vi "Main v0.4.vi"() -> ()   [LabVIEW 2017]
doc: "This template is for the Queued Message Handler design pattern.\n\nThe Event Handling Loop generates messages based on user interface actions.\n\nThe Message Handling Loop processes messages generated by the Event Handling Loop, or by other messages. The messages are string values, so new messages can be added easily to the Message Cases case structure in the Message Handling Loop. Each message cluster can also provide an optional value for Message Data, which is a variant that can be converted to whatever message-specific data is required."
uses:
  Controls/Main Tabs.ctl
  Controls/Auto.ctl
  RT/Controls/Auto Delays.ctl
  RT/Controls/Auto Times.ctl
  <userlib>/SESL Controls/refresh ES.ctl
  Controls/UI Data.ctl
  support/Message Queue/Enqueue Message (Single).vi
  <vilib>/Utility/error.llb/Error Cluster From Error Code.vi
  <vilib>/ErrorRing/Error Ring.xnode
  support/Message Queue/Message Queue.lvlib
  support/User Event - Stop/User Event - Stop.lvlib
panel:
  in  "Enable Reject?":bool
  out "Date-Time":string caption="Dip-Tube Assembly Automation (HMI) v0.4"
  out "Main Tab":T1
  in  "Autocycle":T2
  in  "Manual":bool
  in  "Parameters":bool
  in  "Maintenance":bool
  in  "Save Para":bool
  in  "Home Para":bool
  in  "ParaTab":T3(tab)
  in  "StopperRearDelay":dbl format="%#.2f"
  in  "StopperFrontDelay":dbl format="%#.2f"
  in  "MaxAlarms":dbl caption="Max Alarms in 1 Minute" format="%#.2f"
  in  "MaxConsecutive":dbl caption="Max Consecutive Alarms" format="%#.2f"
  in  "Gate Close Delay":dbl format="%#.2f"
  in  "Gate Open Delay":dbl format="%#.2f"
  in  "BF Off Delay":dbl format="%#.2f"
  in  "BF On Delay":dbl format="%#.2f"
  in  "DelayAfterReject":dbl format="%#.2f"
  in  "MeasurementTime":dbl format="%#.2f"
  in  "DelayAfterMesFront":dbl format="%#.2f"
  in  "DelayAfterCut":dbl format="%#.2f"
  in  "DelayAfterCutClamp":dbl format="%#.2f"
  in  "DelayAfterInsClamp":dbl format="%#.2f"
  in  "DelayToClose":dbl format="%#.2f"
  in  "DelayToOpen":dbl format="%#.2f"
  in  "DelayAfterInsertion":dbl format="%#.2f"
  in  "DelayBeforeInsertion":dbl format="%#.2f"
  in  "AgitatorUpTime":dbl format="%#.2f"
  in  "AgitatorDownTime":dbl format="%#.2f"
  in  "Toggle Motor":bool
  in  "Continuous?":T4
  in  "Enable Measure?":bool
  in  "Enable Index?":bool
  in  "Enable PF?":bool
  in  "Auto Delays":T5={"Agitator Delays"=[1000], "TF Delays"=[1000], "Insertion Delays"=[1000, 1000], "Cutting Delays"=[1000, 1000, 1000], "PF Delays"=[1000], "Measur. Delays"=[1000]}
  in  "Enable Cutting?":bool
  in  "Enable Insertion?":bool
  in  "Run Manual":bool
  in  "Enable TF?":bool
  in  "Home Manual":bool
  out "Status":T7
  out "Measurements":cluster{"1":dbl, "2":dbl, "3":dbl, "4":dbl} {"1" format="%#.2f"; "2" format="%#.2f"; "3" format="%#.2f"; "4" format="%#.2f"}
  in  "All IO":bool
  in  "Stats":bool
  in  "Home AC":bool
  out "Status":string
  out "Count":dbl format="%06.0f"
  out "Count 3":dbl caption="Cycle Time" format="%0.2f"
  out "Count 2":dbl caption="Rejects" format="%06.0f"
  in  "Statuses":string[][](table)
  in  "Exit":bool
  # "Vision Harmony Dip-Tube Assembly Automation"
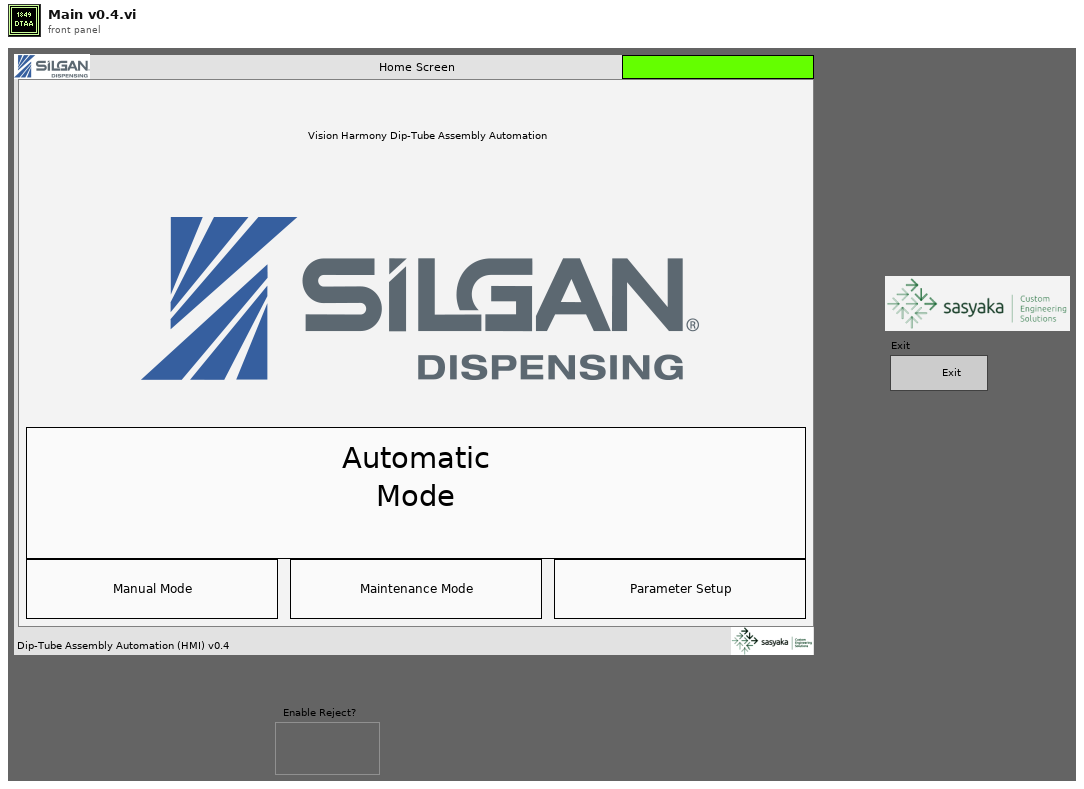
[diagram p1: front panel]
types:
  T1 = typedef "Main Tabs.ctl" = enum32{"Home Screen", "Parameter Setup", "Manual Mode", "Autocycle"}
  T2 = typedef "Auto.ctl" = bool
  T3 = enum32{"General & Indexing", "Bowl Feeder & Pump Conveyor", "Cutting, Measurement & Rejection", "Tube Feeder & Insertion"}
  T4 = typedef "refresh ES.ctl" = bool
  T5 = typedef "Auto Delays.ctl" = cluster{"Agitator Delays":u32[], "TF Delays":u32[], "Insertion Delays":u32[], "Cutting Delays":u32[], "PF Delays":u32[], "Measur. Delays":u32[]}
  T6 = typedef "Auto Times.ctl" = cluster{"Index Time":u32, "TF Time":u32, "Insertion Time":u32, "Cutting Time":u32, "PF Time":u32, "Meas. Time":u32}
  T7 = cluster{"Auto Times":T6, "error out":errorcluster}
  T8 = typedef "UI Data.ctl" = cluster{"Main Tab":refnum<vi>}
  T9 = typedef "Message Queue.lvlib/All Message Queues.ctl" = cluster{"UI":refnum<queue>}
  T10 = enum8{"Enabled", "Disabled", "Disabled and Grayed Out"}
  T11 = cluster{"Auto Times":T6, "Measurements":cluster{"1":dbl, "2":dbl, "3":dbl, "4":dbl}, "error out":errorcluster}
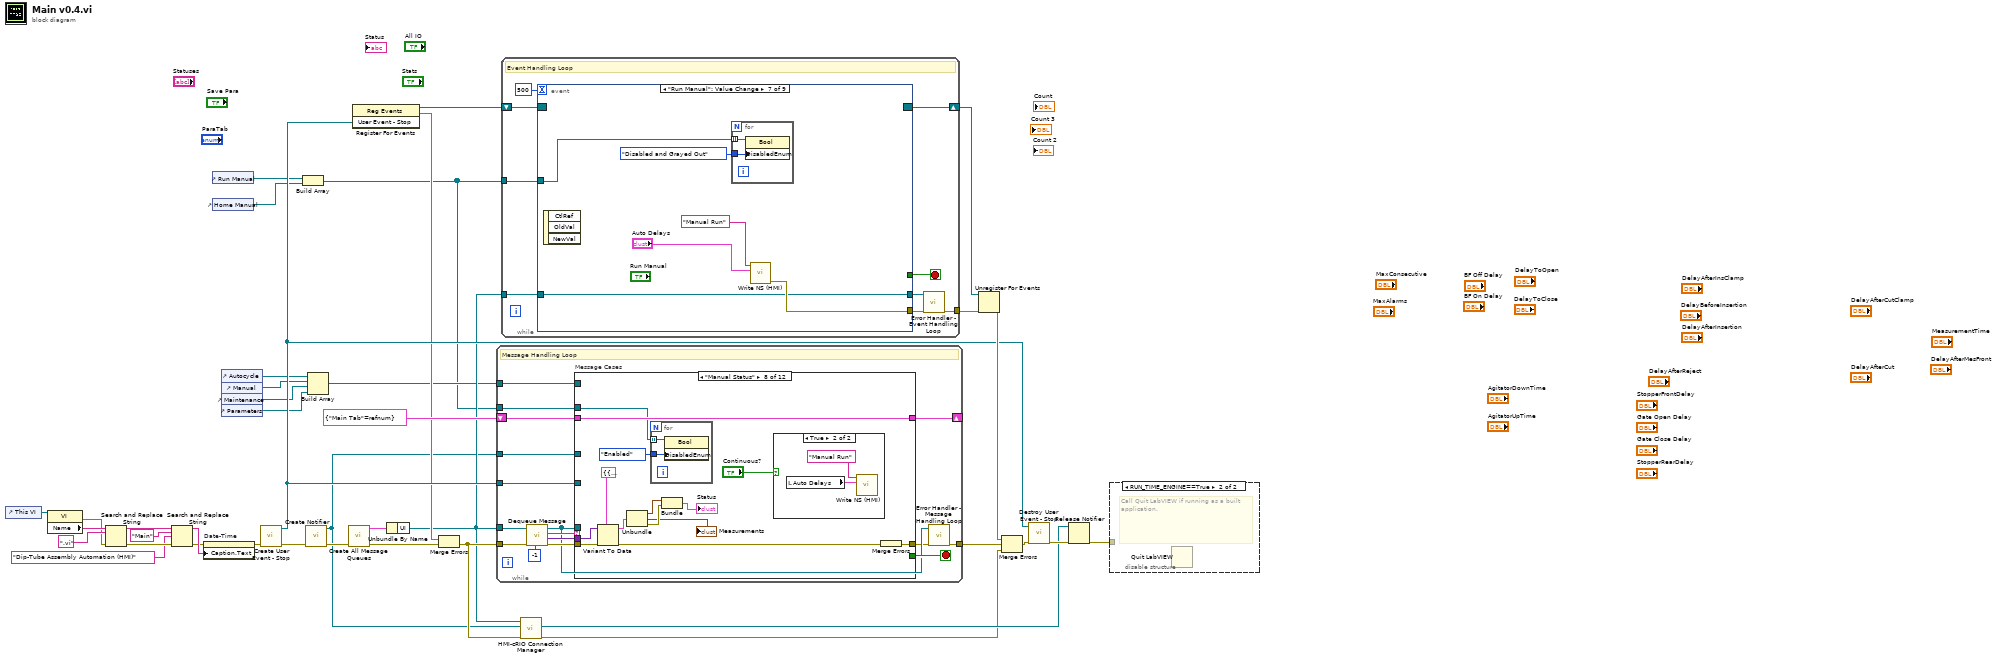
[diagram p0: block diagram]
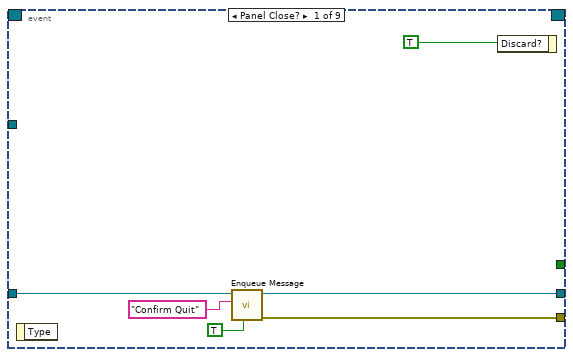
[diagram p2: hidden frame]
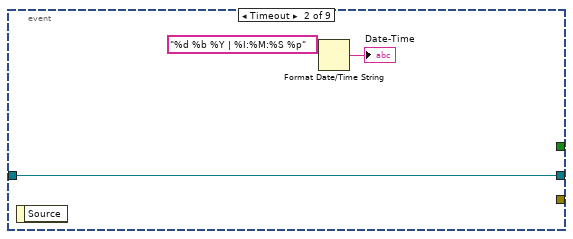
[diagram p3: hidden frame]
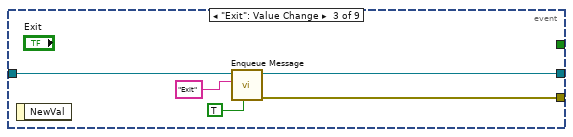
[diagram p4: hidden frame]
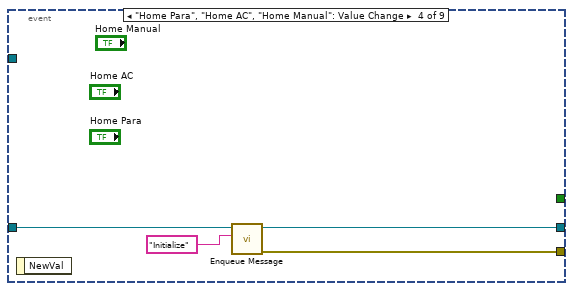
[diagram p5: hidden frame]
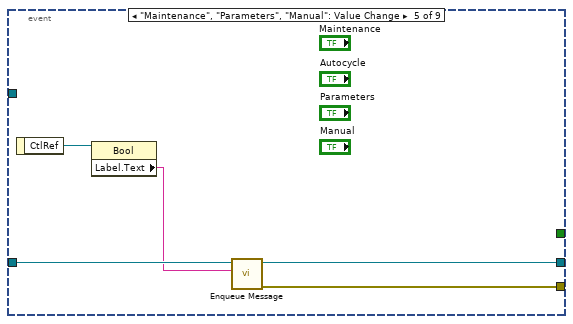
[diagram p6: hidden frame]
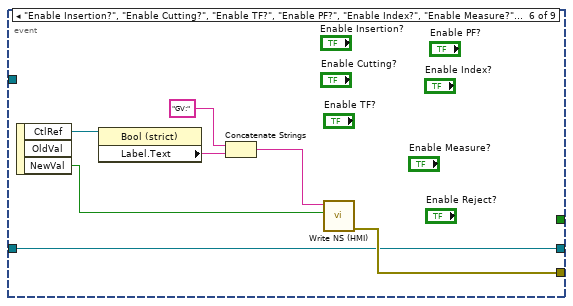
[diagram p7: hidden frame]
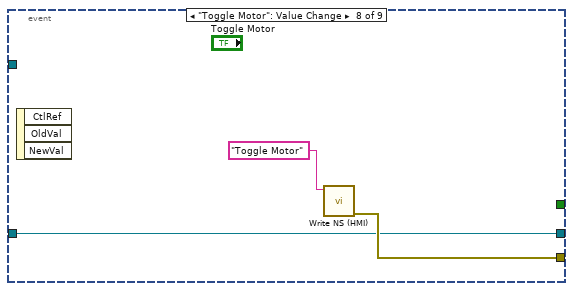
[diagram p8: hidden frame]
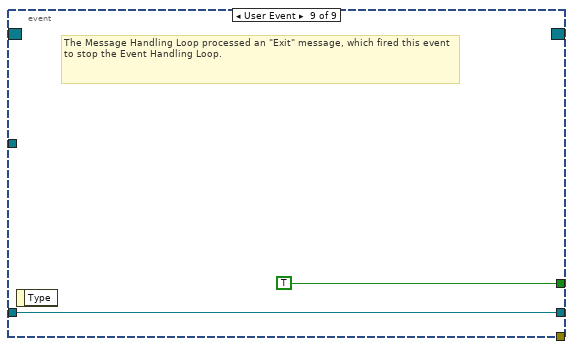
[diagram p9: hidden frame]
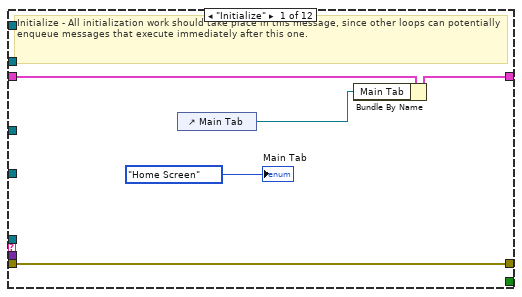
[diagram p10: hidden frame]
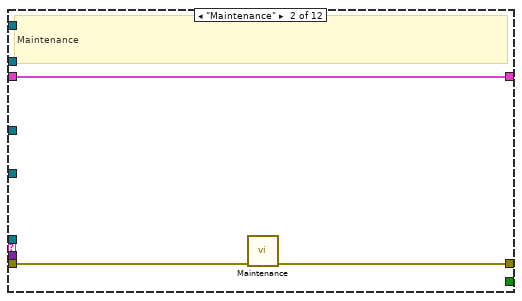
[diagram p11: hidden frame]
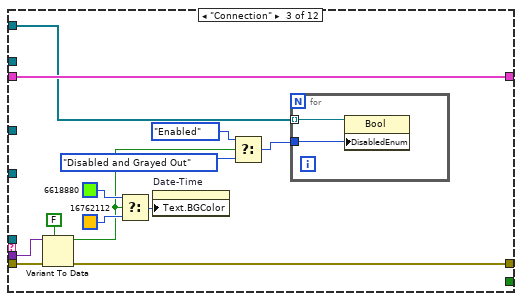
[diagram p12: hidden frame]
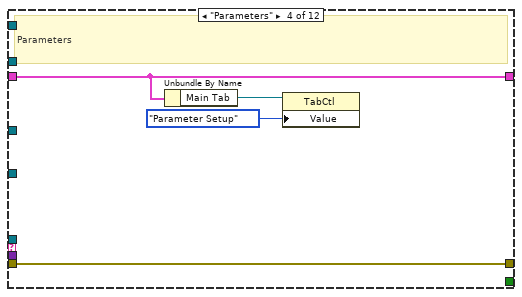
[diagram p13: hidden frame]
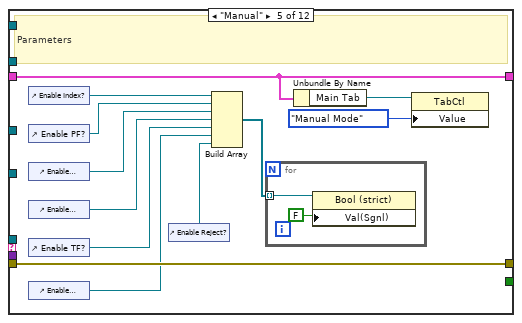
[diagram p14: hidden frame]
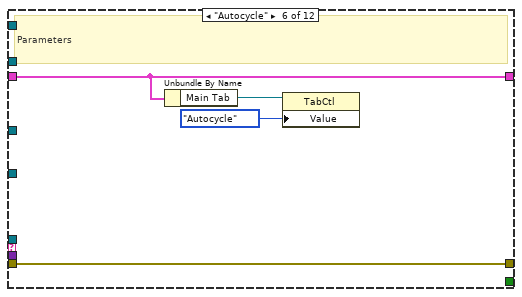
[diagram p15: hidden frame]
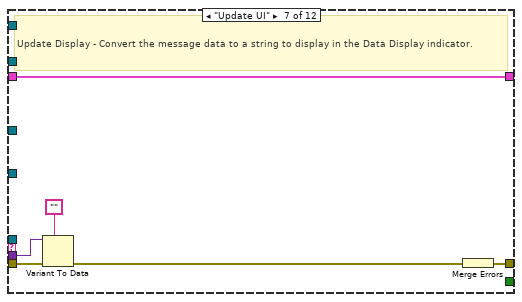
[diagram p16: hidden frame]
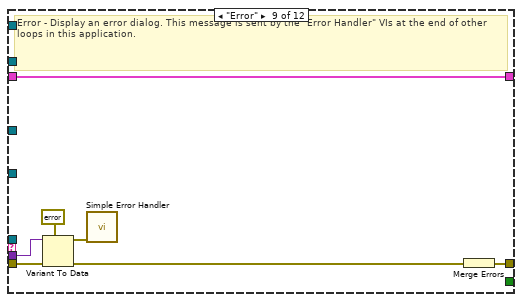
[diagram p18: hidden frame]
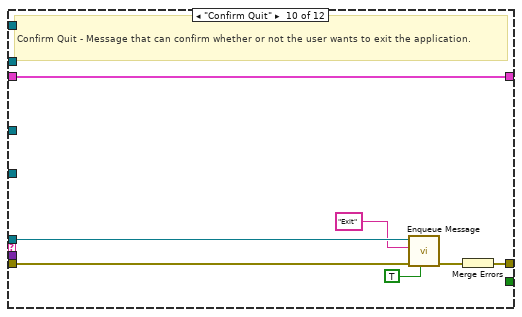
[diagram p19: hidden frame]
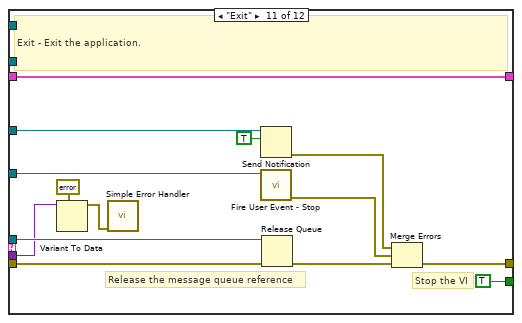
[diagram p20: hidden frame]
diagram:
  n1 = control-ref of="This VI"() -> (w8:refnum<vi>)
  n2 = property class="VI"(reference=w8) -> (error out=w7:errorcluster, "Name"=w14:string)  [unwired: 1 in, 1 out]
  n3 = Search and Replace String(input string=w14, search string=".vi", error in=w7) -> (result string=w12:string, error out=w11:errorcluster)  [unwired: 5 in, 2 out]
  n4 = Search and Replace String(input string=w12, search string="Main", replace string="Dip-Tube Assembly Automation (HMI)" ("replace string (\"\")"), error in=w11) -> (result string=w6:string, error out=w5:errorcluster)  [unwired: 4 in, 2 out]
  n5 = property on="Date-Time" class="Str"(error in=w5, "Caption.Text"=w6) -> (error out=w4:errorcluster)  [unwired: 1 in, 1 out]
  n6 = control-ref of="Run Manual"() -> (w3:refnum<vi>)
  n7 = control-ref of="Home Manual"() -> (w2:refnum<vi>)
  n8 = control-ref of="Autocycle"() -> (w19:refnum<vi>)
  n9 = control-ref of="Manual"() -> (w18:refnum<vi>)
  n10 = control-ref of="Maintenance"() -> (w17:refnum<vi>)
  n11 = control-ref of="Parameters"() -> (w16:refnum<vi>)
  n12 = call "Create User Event - Stop.vi"("error in (no error)"=w4) -> ("error out"=w26:errorcluster, "User Event - Stop"=w30:refnum<user-event>)  [unwired: 9 in]
  n13 = Build Array(w3, w2) -> (w1:refnum<vi>[])
  n14 = call "Create Notifier.vi"("error in (no error)"=w26) -> ("error out"=w25:errorcluster, "notifier out"=w20:refnum<notifier>)  [unwired: 9 in]
  n15 = Build Array(w19, w18, w17, w16) -> (w15:refnum<vi>[])
  n16 = call "Create All Message Queues.vi"("error in (no error)"=w25) -> ("error out"=w39:errorcluster, "Message Queues out"=w38:T9)  [unwired: 9 in]
  n17 = register-events(w30) -> (reference out=w31:refnum<event-registration>, error out=w29:errorcluster)  [unwired: 2 in]
  n18 = Unbundle By Name(w38) -> ("UI"=w27:refnum<queue>)
  n19 = Merge Errors(w29, w39) -> (w28:errorcluster)
  n20 = while {
    tunnel: w27 -> [w47]
    shift-right: [w54] -> _
    shift-left: T8 {"Main Tab"=refnum} ("Data Cluster") -> [w55]
    tunnel: w30 -> [w52]
    tunnel: w28 -> [w51]
    tunnel: [w45] -> w37
    tunnel: w20 -> [w42]
    tunnel: w15 -> [w41]
    tunnel: w1 -> [w40]
    stop <- w53 stop-if-true
    # "Message Handling Loop"
    n21 = call "Dequeue Message.vi"("timeout"=-1, "error in (no error)"=w51, "Message Queue"=w47) -> ("error out"=w50:errorcluster, "Message Data"=w48:variant, "Message"=w49:string, "dup Message Queue"=w46:refnum<queue>)  [unwired: 5 in]
    n22 = case "Message Cases" shown="\"Manual Status\"" w49 {
      selector: w49 -> [_ _ _ _ _ _ _ _ _ _ _ w153]
      tunnel: w46 -> [_ _ _ _ _ _ _ _ _ w134 w152 _]
      tunnel: w50 -> [w60 w62 w74 w82 w94 w100 w104 w118 w131 w138 w145 _]
      tunnel: [w60 w61 w73 w82 w94 w100 w105 w119 w125 w136 w148 w154] -> w44
      tunnel: w55 -> [w59 w63 w76 w81 w93 w99 w106 w120 w130 w137 w151 w155]
      tunnel: [w58 w63 w76 w81 w93 w99 w106 w120 w130 w137 w151 w155] -> w54
      tunnel: [_ _ _ _ _ _ _ _ _ _ TRUE _] -> w53
      tunnel: w48 -> [_ _ w72 _ _ _ w103 w117 w129 _ w142 _]
      tunnel: w52 -> [_ _ _ _ _ _ _ _ _ _ w147 _]
      tunnel: w42 -> [_ _ _ _ _ _ _ _ _ _ w141 _]
      tunnel: w41 -> [_ _ w68 _ _ _ _ _ _ _ _ _]
      tunnel: w40 -> [_ _ _ _ _ _ _ w114 _ _ _ _]
      frame "Initialize" {
        # "Initialize - All initialization work should take place in this message, since other loops can potentially enqueue messages that execute immediately after this one."
        n23 = control-ref of="Main Tab"() -> (w57:refnum<vi>)
        n24 = Bundle By Name(cluster=w59, "Main Tab"=w57) -> (w58:T8)
        "Main Tab" <- Main_Tabs."Home Screen" ("Main Tab")
      }
      frame "Maintenance" {
        # "Maintenance"
        n25 = call "Maintenance.vi"("Error In"=w62) -> ("Error out"=w61:errorcluster)  [unwired: 10 in]
      }
      frame "Connection" {
        n26 = Variant To Data(error in=w74, type=FALSE, Variant=w72) -> (data=w67:bool, error out=w73:errorcluster)
        n27 = Select(t=u32 6618880 ("Text.Text Colors:BG Color"), s=w67, f=u32 16762112 ("Text.Text Colors:BG Color")) -> (s? t:f=w69:u32)
        n28 = property on="Date-Time" class="Str"("Text.BGColor"=w69) -> ()  [unwired: 2 in, 2 out]
        n29 = Select(t=T10."Enabled" ("Disabled"), s=w67, f=T10."Disabled and Grayed Out") -> (s? t:f=w65:T10)
        n30 = for {
          tunnel: w68 -> [w78] mode=indexing
          tunnel: w65 -> [w77]
          n31 = property class="Bool"(reference=w78, "DisabledEnum"=w77) -> ()  [unwired: 1 in, 2 out]
        }
      }
      frame "Parameters" {
        # "Parameters"
        n32 = Unbundle By Name(w81) -> ("Main Tab"=w80:refnum<vi>)
        n33 = property class="TabCtl"(reference=w80, "Value"=Main_Tabs."Parameter Setup" ("Main Tab")) -> ()  [unwired: 1 in, 2 out]
      }
      frame "Manual" {
        # "Parameters"
        n34 = control-ref of="Enable Index?"() -> (w90:refnum<vi>)
        n35 = control-ref of="Enable PF?"() -> (w89:refnum<vi>)
        n36 = control-ref of="Enable Cutting?"() -> (w88:refnum<vi>)
        n37 = control-ref of="Enable Insertion?"() -> (w87:refnum<vi>)
        n38 = control-ref of="Enable TF?"() -> (w86:refnum<vi>)
        n39 = control-ref of="Enable Measure?"() -> (w84:refnum<vi>)
        n40 = control-ref of="Enable Reject?"() -> (w83:refnum<vi>)
        n41 = Build Array(w90, w89, w88, w87, w86, w84, w83) -> (w85:refnum<vi>[])
        n42 = for {
          tunnel: w85 -> [w96] mode=indexing
          n43 = property class="Bool (strict)"(reference=w96, "Val(Sgnl)"=FALSE ("Value (Signaling)")) -> ()  [unwired: 1 in, 2 out]
        }
        n44 = Unbundle By Name(w93) -> ("Main Tab"=w92:refnum<vi>)
        n45 = property class="TabCtl"(reference=w92, "Value"=Main_Tabs."Manual Mode" ("Main Tab")) -> ()  [unwired: 1 in, 2 out]
      }
      frame "Autocycle" {
        # "Parameters"
        n46 = Unbundle By Name(w99) -> ("Main Tab"=w98:refnum<vi>)
        n47 = property class="TabCtl"(reference=w98, "Value"=Main_Tabs."Autocycle" ("Main Tab")) -> ()  [unwired: 1 in, 2 out]
      }
      frame "Update UI" {
        # "Update Display - Convert the message data to a string to display in the Data Display indicator."
        n48 = Variant To Data(error in=w104, type="", Variant=w103) -> (error out=w101:errorcluster)  [unwired: 1 out]
        n49 = Merge Errors(w101) -> (w105:errorcluster)
      }
      frame "Manual Status" {
        n50 = Variant To Data(error in=w118, type=T11 {"Auto Times"={"Index Time"=0, "TF Time"=0, "Insertion Time"=0, "Cutting Time"=0, "PF Time"=0, "Meas. Time"=0}, "Measurements"={"1"=0.0, "2"=0.0, "3"=0.0, "4"=0.0}, "error out"={"status"=FALSE, "code"=0, "source"=""}} ("cluster"), Variant=w117) -> (data=w112:T11, error out=w116:errorcluster)
        n51 = Unbundle(w112) -> ("Auto Times"=w111:T6, "Measurements"=→"Measurements":cluster{"1":dbl, "2":dbl, "3":dbl, "4":dbl}, "error out"=w110:errorcluster)
        n52 = for {
          tunnel: w114 -> [w124] mode=indexing
          tunnel: T10."Enabled" ("Disabled") -> [w123]
          n53 = property class="Bool"(reference=w124, "DisabledEnum"=w123) -> ()  [unwired: 1 in, 2 out]
        }
        n54 = Bundle("Auto Times"=w111, "error out"=w110) -> (→"Status":T7)  [unwired: 1 in]
        n55 = case shown="True" "Continuous?" {
          frame False {
          }
          frame True {
            n56 = local read "Auto Delays"() -> (w121:T5)
            n57 = call "Write NS (HMI).vi"("Message Data"=w121, "Message"="Manual Run") -> ()  [unwired: 9 in, 1 out]
          }
        }
        n58 = Merge Errors(w116) -> (w119:errorcluster)
      }
      frame "Error" {
        # "Error - Display an error dialog. This message is sent by the \"Error Handler\" VIs at the end of other loops in this application."
        n59 = Variant To Data(error in=w131, type=errorcluster {"status"=FALSE, "code"=0, "source"=""} ("error constant"), Variant=w129) -> (data=w127:errorcluster, error out=w126:errorcluster)
        n60 = call <vilib>:"Simple Error Handler.vi"("error in (no error)"=w127) -> ()  [unwired: 4 in, 5 out]
        n61 = Merge Errors(w126) -> (w125:errorcluster)
      }
      frame "Confirm Quit" {
        # "Confirm Quit - Message that can confirm whether or not the user wants to exit the application."
        n62 = call-poly "Enqueue Message.vi"("Priority Message? (F)"=TRUE, "error in (no error)"=w138, "Message"="Exit", "Message Queue"=w134) -> ("error out"=w135:errorcluster)  [unwired: 6 in, 1 out]
        n63 = Merge Errors(w135) -> (w136:errorcluster)
      }
      frame "Exit" {
        # "Stop the VI"
        # "Release the message queue reference"
        # "Exit - Exit the application."
        n64 = Variant To Data(type=errorcluster {"status"=FALSE, "code"=0, "source"=""} ("error constant"), Variant=w142) -> (data=w143:errorcluster)  [unwired: 1 in, 1 out]
        n65 = call <vilib>:"Simple Error Handler.vi"("error in (no error)"=w143) -> ()  [unwired: 4 in, 5 out]
        n66 = Send Notification(notification=TRUE, notifier=w141) -> (error out=w139:errorcluster)  [unwired: 1 in, 1 out]
        n67 = call "Fire User Event - Stop.vi"("User Event - Stop"=w147) -> ("error out"=w146:errorcluster)  [unwired: 10 in]
        n68 = Release Queue(queue=w152, error in (no error)=w145) -> (error out=w149:errorcluster)  [unwired: 1 in, 2 out]
        n69 = Merge Errors(w139, w146, w149) -> (w148:errorcluster)
      }
      frame Default {
        # "'Default' case only runs if there is a message that isn't defined in any of the other cases.  Output a programming error."
        n70 = xnode "Error Ring"("parameter 0"=w153) -> ("error out"=w154:errorcluster)
      }
    }
    n71 = call "Error Handler - Message Handling Loop.vi"("error in (no error)"=w44, "Message Queue"=w46) -> ("dup error in"=w45:errorcluster)  [unwired: 8 in, 1 out]
  }
  n72 = while {
    tunnel: w27 -> [w171]
    shift-right: [w169] -> w34
    shift-left: w31 -> [w170]
    tunnel: [w165] -> w32
    tunnel: w1 -> [w163]
    stop <- w167 stop-if-true
    # "Event Handling Loop"
    n73 = event shown="[6] \"Run Manual\": Value Change" {
      selector: w170 -> [_ _ _ _ _ _ _ _ _]
      dyn-events: [_ _ _ _ _ _ _ _ _] -> w169
      timeout: 500 -> [_ _ _ _ _ _ _ _ _]
      tunnel: [_ _ _ _ _ _ _ _ TRUE ("Discard?")] -> w167
      tunnel: w171 -> [w176 w180 w185 w189 w194 w199 w206 w211 w214]
      tunnel: [w175 _ w184 w188 w193 w200 w207 w212 _] -> w168
      tunnel: [w174 w180 w183 w187 w192 w199 w206 w211 w214] -> w166
      tunnel: w163 -> [_ _ _ _ _ _ w203 _ _]
      event Panel Close? {
        n74 = event-data() -> ()  [unwired: 1 in, 1 out]
        n75 = call-poly "Enqueue Message.vi"("Priority Message? (F)"=TRUE, "Message"="Confirm Quit", "Message Queue"=w176) -> ("error out"=w175:errorcluster, "dup Message Queue"=w174:refnum<queue>)  [unwired: 7 in]
        n76 = event-data("Discard?"=TRUE) -> ()  [unwired: 1 in, 1 out]
      }
      event Timeout {
        n77 = event-data() -> ()  [unwired: 1 in, 1 out]
        n78 = Format Date/Time String(time format string (%c)="%d %b %Y | %I:%M:%S %p") -> (date/time string=→"Date-Time":string)  [unwired: 2 in]
      }
      event "Exit": Value Change {
        n79 = event-data() -> ()  [unwired: 1 in, 1 out]
        n80 = call-poly "Enqueue Message.vi"("Priority Message? (F)"=TRUE, "Message"="Exit", "Message Queue"=w185) -> ("error out"=w184:errorcluster, "dup Message Queue"=w183:refnum<queue>)  [unwired: 7 in]
      }
      event "Home Para", "Home AC", "Home Manual": Value Change {
        n81 = event-data() -> ()  [unwired: 1 in, 1 out]
        n82 = call-poly "Enqueue Message.vi"("Message"="Initialize", "Message Queue"=w189) -> ("error out"=w188:errorcluster, "dup Message Queue"=w187:refnum<queue>)  [unwired: 8 in]
      }
      event "Maintenance", "Parameters", "Manual": Value Change {
        n83 = event-data() -> ("CtlRef"=w191:refnum<vi>)  [unwired: 1 in]
        n84 = property class="Bool"(reference=w191) -> ("Label.Text"=w190:string)  [unwired: 1 in, 2 out]
        n85 = call-poly "Enqueue Message.vi"("Message"=w190, "Message Queue"=w194) -> ("error out"=w193:errorcluster, "dup Message Queue"=w192:refnum<queue>)  [unwired: 8 in]
      }
      event "Enable Insertion?", "Enable Cutting?", "Enable TF?", "Enable PF?", "Enable Index?", "Enable Measure?", "Enable Reject?": Value Change {
        n86 = event-data() -> ("CtlRef"=w201:refnum<vi>, "NewVal"=w195:bool)  [unwired: 1 in, 1 out]
        n87 = property class="Bool (strict)"(reference=w201) -> ("Label.Text"=w198:string)  [unwired: 1 in, 2 out]
        n88 = Concatenate Strings("GV:" ("string"), w198) -> (w196:string)
        n89 = call "Write NS (HMI).vi"("Message Data"=w195, "Message"=w196) -> ("error out"=w200:errorcluster)  [unwired: 9 in]
      }
      event "Run Manual": Value Change {
        n90 = event-data() -> ()  [unwired: 1 in, 3 out]
        n91 = for {
          tunnel: w203 -> [w209] mode=indexing
          tunnel: T10."Disabled and Grayed Out" ("Disabled") -> [w208]
          n92 = property class="Bool"(reference=w209, "DisabledEnum"=w208) -> ()  [unwired: 1 in, 2 out]
        }
        n93 = call "Write NS (HMI).vi"("Message Data"="Auto Delays", "Message"="Manual Run") -> ("error out"=w207:errorcluster)  [unwired: 9 in]
      }
      event "Toggle Motor": Value Change {
        n94 = event-data() -> ()  [unwired: 1 in, 3 out]
        n95 = call "Write NS (HMI).vi"("Message"="Toggle Motor") -> ("error out"=w212:errorcluster)  [unwired: 10 in]
      }
      event User Event {
        # "The Message Handling Loop processed an \"Exit\" message, which fired this event to stop the Event Handling Loop."
        n96 = event-data() -> ()  [unwired: 1 in, 1 out]
      }
    }
    n97 = call "Error Handler - Event Handling Loop.vi"("error in (no error)"=w168, "Message Queue"=w166) -> ("dup error in"=w165:errorcluster)  [unwired: 8 in, 1 out]
  }
  n98 = call "HMI-cRIO Connection Manager.vi"("error in"=w28, "notifier in"=w20, "Queue in"=w27) -> ("error out"=w21:errorcluster, "Notifier out"=w22:refnum<notifier>)  [unwired: 7 in]
  n99 = Unregister For Events(event registration refnum=w34, error in=w32) -> (error out=w35:errorcluster)
  n100 = Merge Errors(w35, w37, w21) -> (w36:errorcluster)
  n101 = call "Destroy User Event - Stop.vi"("error in (no error)"=w36, "User Event - Stop"=w30) -> ("error out"=w24:errorcluster)  [unwired: 9 in]
  n102 = Release Notifier(notifier=w22, error in (no error)=w24) -> (error out=w23:errorcluster)  [unwired: 1 in, 2 out]
  n103 = disable-structure shown="RUN_TIME_ENGINE==True" {
    disable-tunnel: w23 -> [_ _]
    frame condition #0 (active) {
    }
    frame condition #1 {
      # "Call Quit LabVIEW if running as a built application."
      n104 = Quit LabVIEW() -> ()  [unwired: 1 in]
    }
  }
